vi "BITMAPFILEHEADER.vi"(11 "Image Dimensions":i32[](array[numeric])) -> (3 "BITMAPFILEHEADER":u8[](array[numeric]))   [LabVIEW 2010]
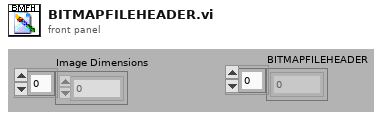
[diagram p1: front panel]
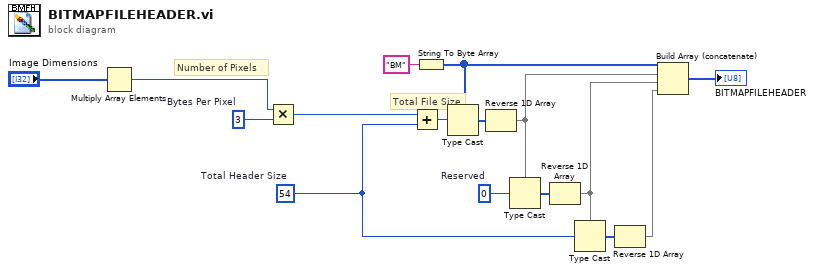
[diagram p0: block diagram]
diagram:
  w16 = 54  # Total Header Size
  w15 = 0  # Reserved
  w10 = 3  # Bytes Per Pixel
  # "Total File Size"
  # "Number of Pixels"
  n1 = Multiply Array Elements(1:"Image Dimensions") -> (0:w13:i32)
  n2 = Multiply(x=w13, y=w10) -> (x*y=w1:i32)
  n3 = Add(x=w1, y=w16) -> (x+y=w8:i32)
  n4 = String To Byte Array(string="BM") -> (unsigned byte array=w9:u8[])
  n5 = Type Cast(type=w9, x=w8) -> (*(type *) &x=w7:u8[])
  n6 = Reverse 1D Array(array=w7) -> (reversed array=w6:u8[])
  n7 = Type Cast(type=w6, x=w15) -> (*(type *) &x=w5:u8[])
  n8 = Reverse 1D Array(array=w5) -> (reversed array=w4:u8[])
  n9 = Type Cast(type=w4, x=w16) -> (*(type *) &x=w2:u8[])
  n10 = Reverse 1D Array(array=w2) -> (reversed array=w3:u8[])
  n11 = Build Array (concatenate)(w9, w6, w4, w3) -> (→"BITMAPFILEHEADER":u8[])
